vi "lsl push chunk ftp.vi"(6 "pushthrough":i32, 7 "timestamp":dbl, 8 "error in (no error)":errorcluster, 9 "data_elements":u32, 10 "data":sgl[][](array[numeric]), 11 "outlet":T1) -> (0 "error out":errorcluster, 2 "function return":i32)   [LabVIEW 2016, in "Lab Streaming Layer.lvlib"]
doc: "extern LIBLSL_C_API int32_t lsl_push_chunk_ftp(lsl_outlet out, const float *data, unsigned long data_elements, double timestamp, int32_t pushthrough);"
uses:
  Lab Streaming Layer.lvlib
  <userlib>/liblsl-LabVIEW/liblsl64.dll
  Custom Controls/lsl_outlet.ctl
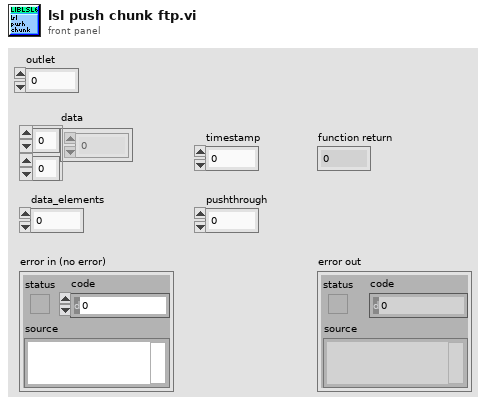
[diagram p1: front panel]
types:
  T1 = typedef "liblsl-LabVIEW.lvlib/lsl_outlet.ctl" = u64
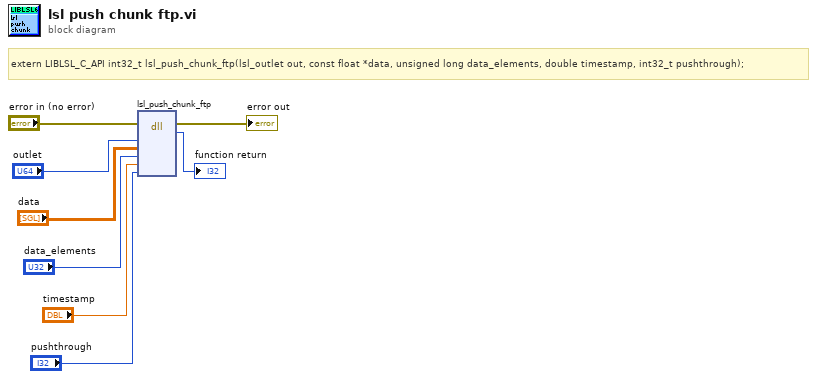
[diagram p0: block diagram]
diagram:
  # "extern LIBLSL_C_API int32_t lsl_push_chunk_ftp(lsl_outlet out, const float *data, unsigned long data_elements, double timestamp, int32_t pushthrough);"
  n1 = dll-call lib="C:/Program Files/National Instruments/LabVIEW 2018/user.lib/liblsl-LabVIEW/liblsl64.*" fn="lsl_push_chunk_ftp"(error in="error in (no error)", "out"="outlet", "data"="data", "data_elements"="data_elements", "timestamp"="timestamp", "pushthrough"="pushthrough") -> (error out=→"error out":errorcluster, "return type"=→"function return":i32)  [unwired: 7 in, 1 out]
